vi "RT Loop - Analyze Acceleration_V4.vi"(7 "testing":bool, 8 "error in (no error)":errorcluster, 9 "Acceleration RT FIFO In":T1, 10 "FPGA VI Reference Out 2":refnum<k20>, 11 "Message Queue":refnum<queue>) -> (1 "Acceleration RT FIFO Out":T1)   [LabVIEW 2017]
doc: "Read and analyze acceleration waveform data from FPGA via DMA FIFO. If the acceleration is over the limit, then send the acceleration waveform data to the Log Data Loop."
uses:
  UI Error Handlers/support/Message Queue/Message Cluster.ctl
  controls/Acceleration RT FIFO Reference.ctl
  Globals/Global - All RT Loop Stop.vi
  Globals/Global - Configuration Options.vi
  <vilib>/Utility/error.llb/Error Cluster From Error Code.vi
  <vilib>/rvi/errors/niLvFpgaAdjustHostInterfaceError.vi
  <vilib>/rvi/interface/nirviMethod/nirviMethod.xnode
  <vilib>/FPGAPlugInAG/Dynamic/niLvFpga_ReadFifo_Dynamic.vi
  <vilib>/rvi/errors/niLvFpgaMergeErrorWithErrorCode.vi
  UI Error Handlers/support/Message Queue/Message Queue.lvlib
panel:
  out "x-y":u32
  out "G1 status.G1 trigger":bool
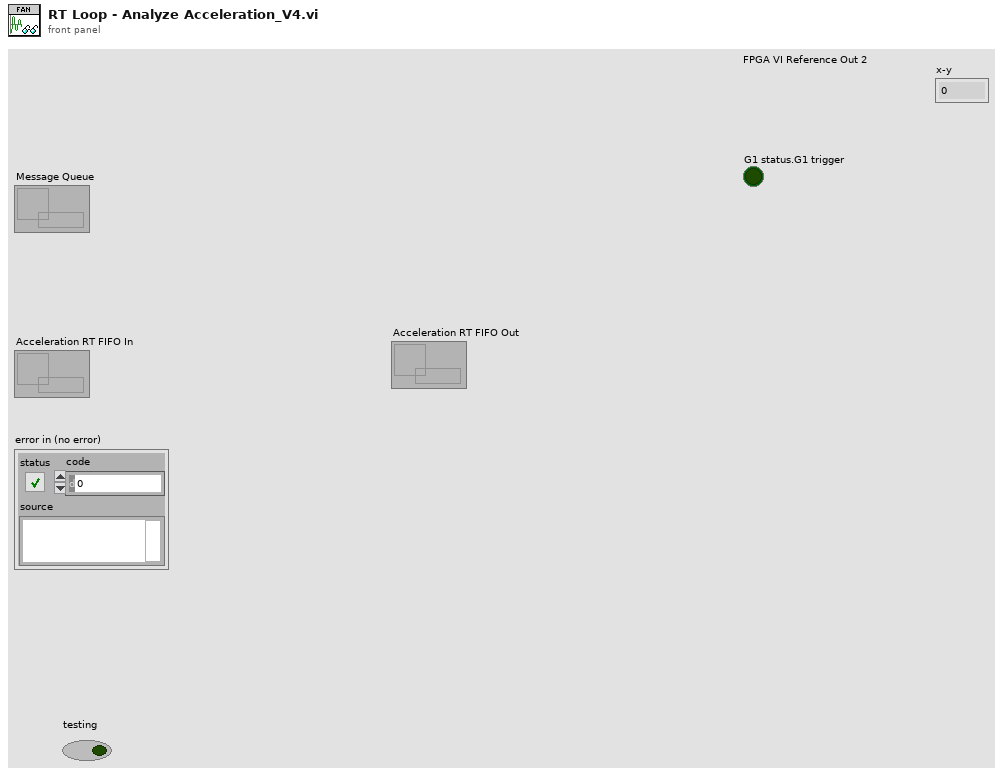
[diagram p1: front panel]
types:
  T1 = typedef "Acceleration RT FIFO Reference.ctl" = refnum<k33>
  T2 = cluster{"Tool data":cluster{"Number of teeth":sgl}, "Cutting data":cluster{"rpm":sgl}, "Limits":cluster{"Magnitude threshold":sgl, "Tolerance":sgl}, "G1 status":cluster{"G1 trigger":bool}}
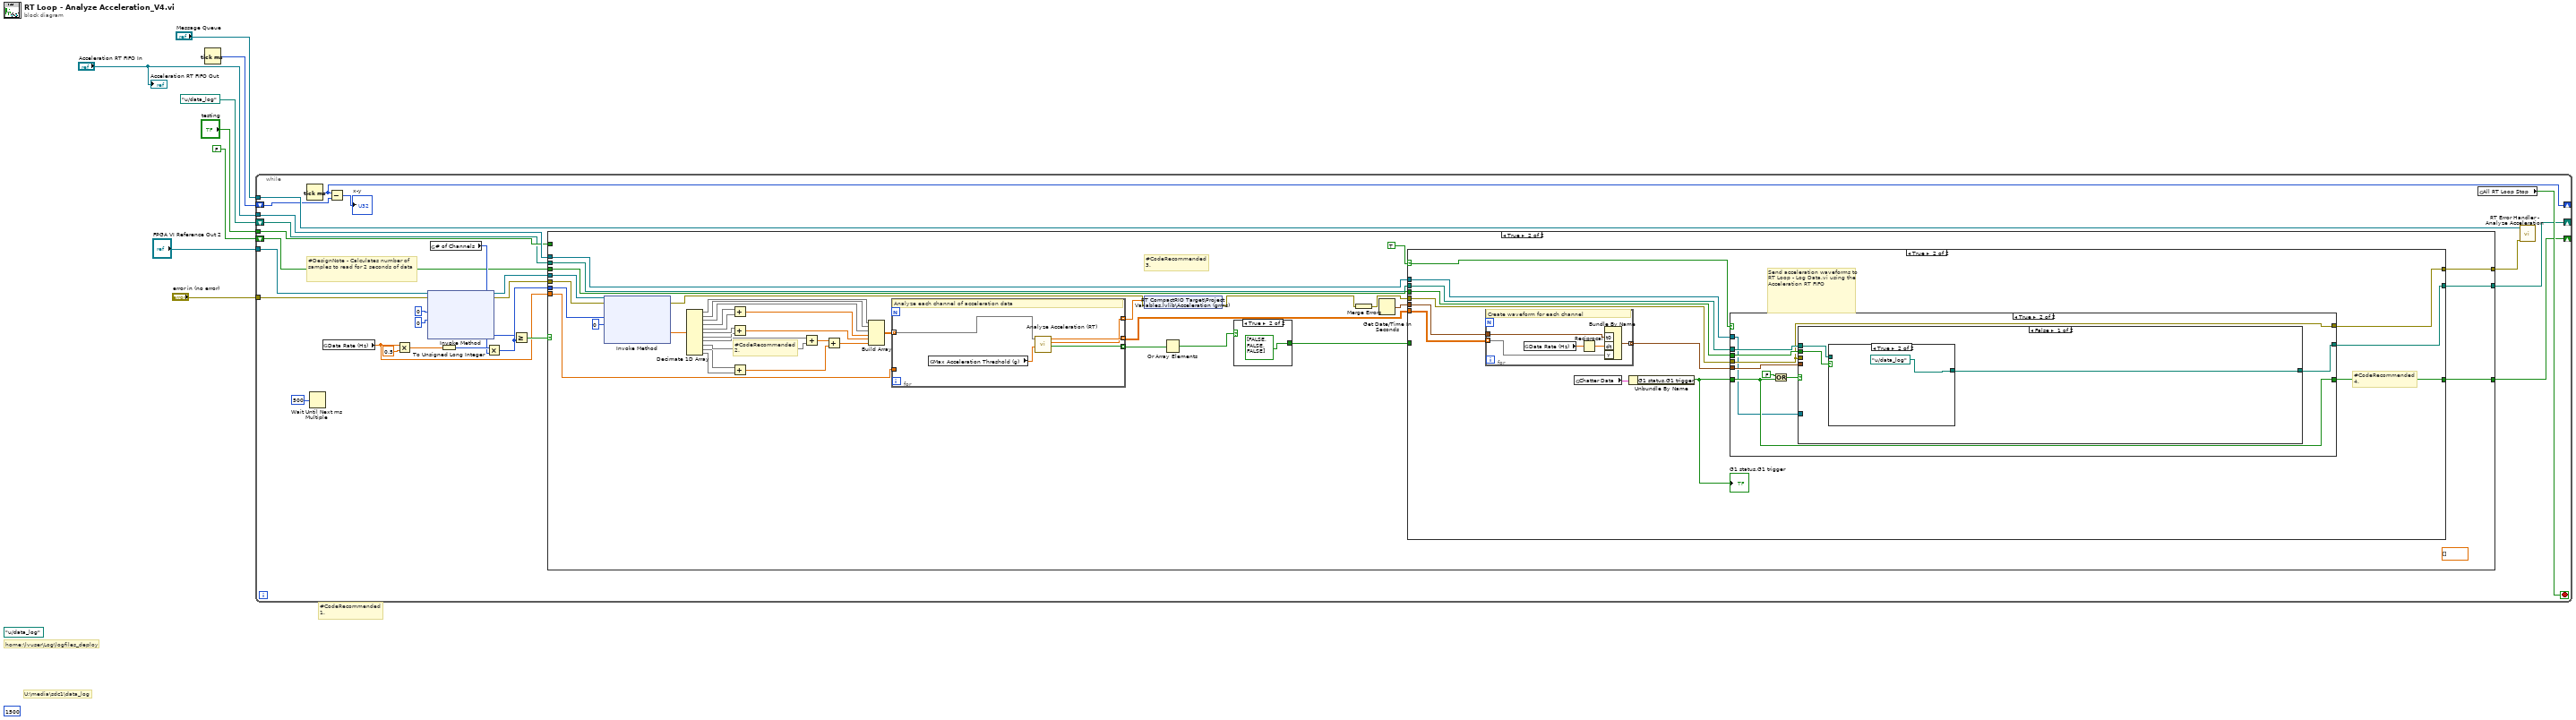
[diagram p0: block diagram]
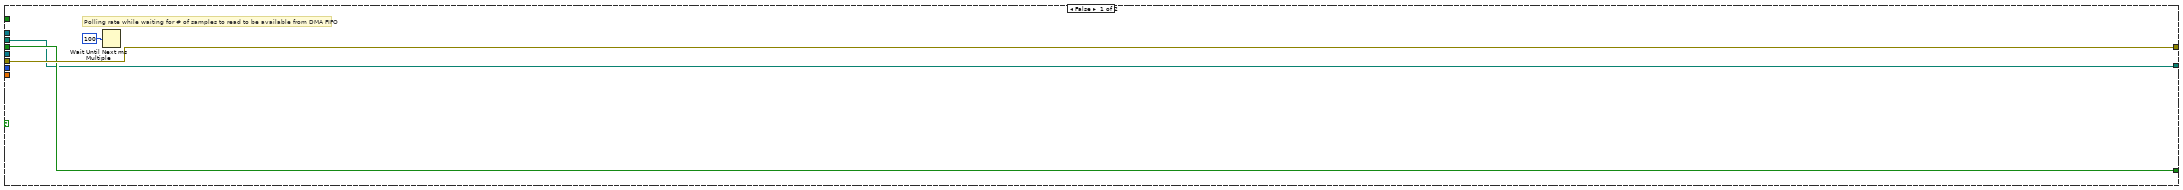
[diagram p2: hidden frame]
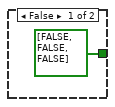
[diagram p3: hidden frame]
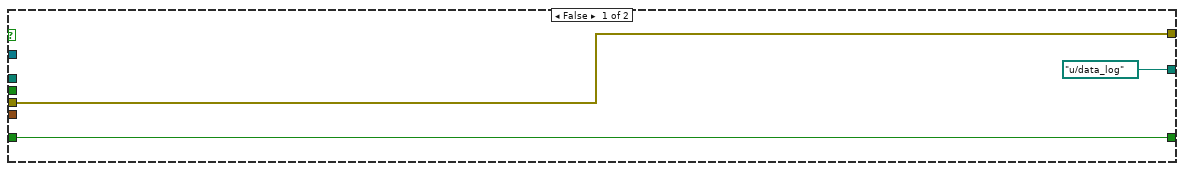
[diagram p5: hidden frame]
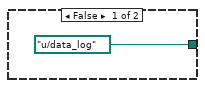
[diagram p6: hidden frame]
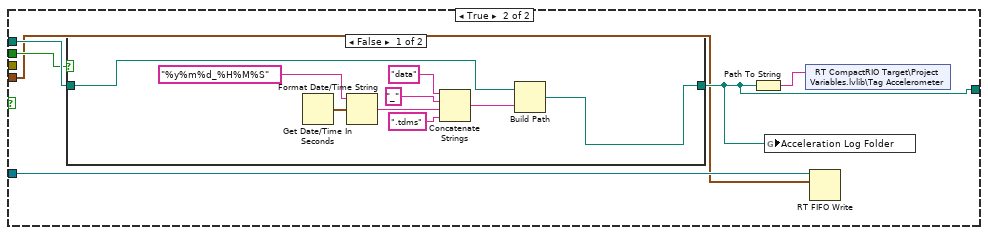
[diagram p7: hidden frame]
diagram:
  (unwired) 1500 ("max queue size (-1, unlimited)")
  (unwired) path "u:/data_log" ("AVI Path")
  # "U:\\media\\sdc1\\data_log"
  # "home:\\lvuser\\Log\\logfiles_deploy"
  # "#CodeRecommended\n1."
  n1 = Tick Count (ms)() -> (millisecond timer value=w2:u32)
  n2 = while {
    tunnel: "FPGA VI Reference Out 2" -> [w35]
    tunnel: "error in (no error)" -> [w34]
    tunnel: "Message Queue" -> [w27]
    tunnel: "Acceleration RT FIFO In" -> [w25]
    tunnel: "testing" -> [w17]
    shift-right: [w14] -> _
    shift-left: path "u:/data_log" ("AVI Path") -> [w13]
    shift-right: [w16] -> _
    shift-left: FALSE -> [w15]
    shift-right: [w11] -> _
    shift-left: w2 -> [w12]
    stop <- w28 stop-if-true
    # "#DesignNote - Calculates number of samples to read for 2 seconds of data"
    n3 = Tick Count (ms)() -> (millisecond timer value=w11:u32)
    n4 = Wait Until Next ms Multiple(millisecond multiple=u32 500) -> ()  [unwired: 1 out]
    n5 = global read "Global - Configuration Options.vi" "Data Rate (Hz)"() -> (w19:dbl)
    n6 = Subtract(x=w11, y=w12) -> (x-y=→"x-y":u32)
    n7 = Multiply(x=w19, y=0.5) -> (x*y=w23:dbl)
    n8 = xnode "Invoke Method"("FPGA VI Reference In"=w35, "error in"=w34, "Number of Elements"=u32 0, "Timeout (ms)"=0) -> ("FPGA VI Reference Out"=w31:refnum<k20>, "error out"=w30:errorcluster, "Elements Remaining"=w18:u32)  [unwired: 1 out]
    n9 = global read "Global - Configuration Options.vi" "# of Channels"() -> (w20:u32)
    n10 = To Unsigned Long Integer(number=w23) -> (unsigned 32bit integer=w22:u32)
    n11 = Multiply(x=w22, y=w20) -> (x*y=w21:u32)
    n12 = Greater Or Equal?(x=w18, y=w21) -> (x >= y?=w29:bool)
    n13 = case shown="True" w29 {
      tunnel: w31 -> [_ w78]
      tunnel: w30 -> [w39 w77]
      tunnel: [w39 w73] -> w26
      tunnel: w21 -> [_ w76]
      tunnel: w25 -> [_ w71]
      tunnel: w19 -> [_ w68]
      tunnel: w17 -> [_ _]
      tunnel: [w37 w62] -> w16
      tunnel: w15 -> [w37 w61]
      tunnel: [w36 w60] -> w14
      tunnel: w13 -> [w36 w59]
      frame False {
        # "Polling rate while waiting for # of samples to read to be available from DMA FIFO"
        n14 = Wait Until Next ms Multiple(millisecond multiple=u32 100) -> ()  [unwired: 1 out]
      }
      frame True {
        (unwired) dbl[] []
        # "#CodeRecommended\n3."
        # "#CodeRecommended\n2."
        n15 = xnode "Invoke Method"("FPGA VI Reference In"=w78, "error in"=w77, "Number of Elements"=w76, "Timeout (ms)"=0) -> ("error out"=w67:errorcluster, "Data"=w70:sgl[])  [unwired: 2 out]
        n16 = Decimate 1D Array(w70) -> (w56:sgl[], w55:sgl[], w54:sgl[], w53:sgl[], w52:sgl[], w50:sgl[], w49:sgl[], w48:sgl[], w47:sgl[], w46:sgl[], w45:sgl[])
        n17 = Add(x=w53, y=w52) -> (x+y=w51:sgl[])
        n18 = Add(x=w50, y=w49) -> (x+y=w41:sgl[])
        n19 = Add(x=w46, y=w45) -> (x+y=w43:sgl[])
        n20 = Add(x=w48, y=w47) -> (x+y=w44:sgl[])
        n21 = Add(x=w44, y=w43) -> (x+y=w42:sgl[])
        n22 = Build Array(w56, w55, w54, w51, w41, w42) -> (w57:sgl[][])
        n23 = for {
          tunnel: [w85] -> w72 mode=indexing
          tunnel: [w84] -> w69 mode=indexing
          tunnel: [w83] -> w40 mode=indexing
          tunnel: w68 -> [_]
          tunnel: w57 -> [w81] mode=indexing
          # "Analyze each channel of acceleration data"
          n24 = global read "Global - Configuration Options.vi" "Max Acceleration Threshold (g)"() -> (w82:sgl)
          n25 = call "Analyze Acceleration (RT).vi"("Max Instantaneous Acceleration (g)"=w82, "Acceleration Waveform (SGL)"=w81) -> ("Over Limit?"=w85:bool, "Acceleration (grms)"=w83:dbl, "Acceleration Waveform (DBL)"=w84:dbl[])  [unwired: 7 in]
        }
        n26 = shared-variable "RT CompactRIO Target\\Project Variables.lvlib\\Acceleration (grms)"(w40, error in=w67) -> (error out=w66:errorcluster)
        n27 = Or Array Elements(Boolean array=w72) -> (logical OR=w64:bool)
        n28 = case shown="True" w64 {
          tunnel: [bool[] [FALSE, FALSE, FALSE] ("Chatter?") bool[] [FALSE, FALSE, FALSE] ("Chatter?")] -> w63
          frame False {
          }
          frame True {
          }
        }
        n29 = Merge Errors(w66) -> (w65:errorcluster)
        n30 = Get Date/Time In Seconds() -> (seconds since 1Jan1904=w74:timestamp)
        n31 = case shown="True" TRUE {
          selector: TRUE -> [_ w89]
          tunnel: w74 -> [_ w101]
          tunnel: w65 -> [w88 w100]
          tunnel: [w88 w90] -> w73
          tunnel: w71 -> [_ w98]
          tunnel: w69 -> [_ w97]
          tunnel: w63 -> [_ _]
          tunnel: [w87 w95] -> w62
          tunnel: w61 -> [w87 w94]
          tunnel: [w86 w93] -> w60
          tunnel: w59 -> [w86 w91]
          frame False {
          }
          frame True {
            # "#CodeRecommended\n4."
            # "Send acceleration waveforms to RT Loop - Log Data.vi using the Acceleration RT FIFO"
            n32 = for {
              tunnel: w97 -> [w139] mode=indexing
              tunnel: w101 -> [w138]
              tunnel: [w136] -> w99 mode=indexing
              # "Create waveform for each channel"
              n33 = global read "Global - Configuration Options.vi" "Data Rate (Hz)"() -> (w135:dbl)
              n34 = Reciprocal(x=w135) -> (1/x=w137:dbl)
              n35 = Bundle By Name("t0"=w138, "dt"=w137, "Y"=w139) -> (w136:waveform(dbl))  [unwired: 1 in]
            }
            n36 = global read "Global - Configuration Options.vi" "Chatter Data"() -> (w96:T2)
            n37 = Unbundle By Name(w96) -> ("G1 status.G1 trigger"=w92:bool)
            "G1 status.G1 trigger" <- w92
            n38 = case shown="True" w89 {
              tunnel: w100 -> [w104 w106]
              tunnel: w99 -> [_ w107]
              tunnel: w98 -> [_ w105]
              tunnel: w92 -> [w103 w111]
              tunnel: [w103 w111] -> w95
              tunnel: w94 -> [_ w110]
              tunnel: [path "u:/data_log" ("AVI Path") w109] -> w93
              tunnel: w91 -> [_ w108]
              tunnel: [w104 w106] -> w90
              frame False {
              }
              frame True {
                n39 = Or(x=FALSE, y=w111) -> (x .or. y?=w113:bool)
                n40 = case shown="False" w113 {
                  tunnel: w108 -> [w114 w124]
                  tunnel: [w116 w121] -> w109
                  tunnel: w110 -> [w115 w123]
                  tunnel: w107 -> [_ w119]
                  tunnel: w106 -> [_ _]
                  tunnel: w105 -> [_ w120]
                  frame False {
                    n41 = case shown="True" w115 {
                      tunnel: [path "u:/data_log" ("AVI Path") path "u:/data_log" ("AVI Path")] -> w116
                      tunnel: w114 -> [_ _]
                      frame False {
                      }
                      frame True {
                      }
                    }
                  }
                  frame True {
                    n42 = case shown="False" w123 {
                      tunnel: w124 -> [w126 w134]
                      tunnel: [w125 w134] -> w121
                      frame False {
                        n43 = Get Date/Time In Seconds() -> (seconds since 1Jan1904=w129:timestamp)
                        n44 = Format Date/Time String(time format string (%c)="%y%m%d_%H%M%S", seconds (now)=w129) -> (date/time string=w132:string)  [unwired: 1 out]
                        n45 = Concatenate Strings("data" ("string"), "_" ("string"), w132, ".tdms" ("string")) -> (w127:string)
                        n46 = Build Path(base path=w126, name or relative path=w127) -> (appended path=w125:path)
                      }
                      frame True {
                      }
                    }
                    n47 = Path To String(path=w121) -> (string=w122:string)
                    n48 = global write "Global - Configuration Options.vi" "Acceleration Log Folder"(w121) -> ()
                    n49 = shared-variable "RT CompactRIO Target\\Project Variables.lvlib\\Tag Accelerometer"(w122) -> ()  [unwired: 1 in, 1 out]
                    n50 = RT FIFO Write(0:w120, 1:w119) -> ()  [unwired: 3 in, 4 out]
                  }
                }
              }
            }
          }
        }
      }
    }
    n51 = global read "Global - All RT Loop Stop.vi" "All RT Loop Stop"() -> (w28:bool)
    n52 = call "RT Error Handler - Analyze Acceleration.vi"("error in (no error)"=w26, "Message Queue"=w27) -> ()  [unwired: 9 in, 1 out]
  }
  "Acceleration RT FIFO Out" <- "Acceleration RT FIFO In"
